vi "Escribir error en Log.vi"(8 "Error In":errorcluster, 11 "Ruta Log":path) -> (0 "Error Out":errorcluster, 1 "# Errores en queue":i32, 2 "Mensaje Error":string, 3 "Ruta Out":path, 4 "error":bool)   [LabVIEW 2018]
doc: "Este VI lee los errores que hayan sido insertados en la \"Queue Errores\" y los registra en el Log de Errores y Eventos del Software ESA."
uses:
  Global/Error Queue Reference.vi
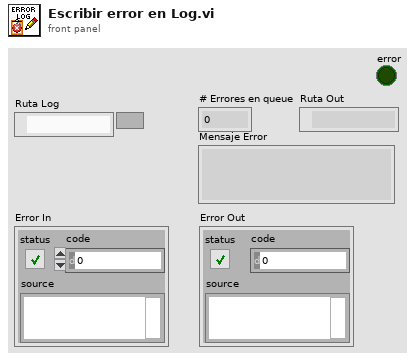
[diagram p1: front panel]
types:
  T1 = enum16{"open", "replace", "create", "open or create", "replace or create", "replace or create with confirmation"}
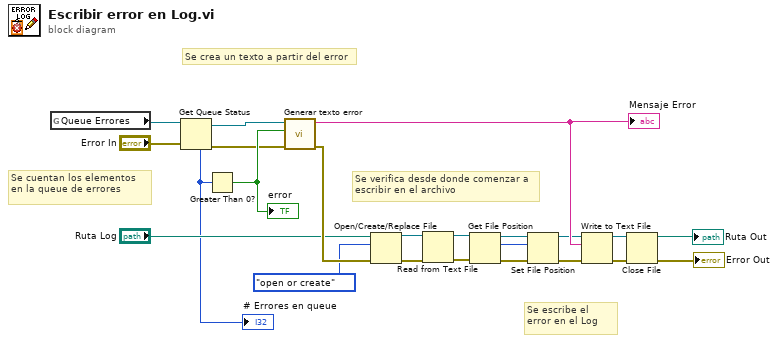
[diagram p0: block diagram]
diagram:
  # "Se escribe el error en el Log"
  # "Se verifica desde donde comenzar a escribir en el archivo"
  # "Se crea un texto a partir del error"
  # "Se cuentan los elementos en la queue de errores"
  n1 = global read "Error Queue Reference.vi" "Queue Errores"() -> (w15:refnum<queue>)
  n2 = Get Queue Status(queue=w15, error in (no error)="Error In") -> (queue out=w17:refnum<queue>, error out=w16:errorcluster, # elements in queue=w13:i32)  [unwired: 1 in, 5 out]
  "# Errores en queue" <- w13
  n3 = Greater Than 0?(x=w13) -> (x > 0?=w18:bool)
  "error" <- w18
  n4 = call "Generar texto error.vi"("Error In"=w16, "Boolean"=w18, "Queue in"=w17) -> ("error out"=w22:errorcluster, "Mensaje Error"=w19:string)  [unwired: 7 in]
  "Mensaje Error" <- w19
  n5 = Open/Create/Replace File(file path (use dialog)="Ruta Log", error in=w22, operation (0:open)=T1."open or create") -> (refnum out=w2:refnum<file>, error out=w5:errorcluster)  [unwired: 3 in, 1 out]
  n6 = Read from Text File(file (use dialog)=w2, error in=w5) -> (refnum out=w3:refnum<file>, error out=w4:errorcluster)  [unwired: 2 in, 2 out]
  n7 = Get File Position(4:w4, 7:w3) -> (0:w10:errorcluster, 2:w6:i64, 3:w9:refnum<file>)
  n8 = Set File Position(offset (in bytes) (0)=w6, refnum=w9, error in=w10) -> (refnum out=w7:refnum<file>, error out=w8:errorcluster)  [unwired: 1 in]
  n9 = Write to Text File(file (use dialog)=w7, text=w19, error in=w8) -> (refnum out=w11:refnum<file>, error out=w12:errorcluster)  [unwired: 1 in, 1 out]
  n10 = Close File(refnum=w11, error in=w12) -> (path=→"Ruta Out":path, error out=→"Error Out":errorcluster)
